vi "Initialize.vi"(8 "error in (no error)":errorcluster) -> (0 "error out":errorcluster, 3 "SGDV FPGA Target":refnum<class "SGDV FPGA Target.lvclass">)   [LabVIEW 2013, in "SGDV_Ctrl_v13_lib.lvlib" / "SGDV FPGA Target.lvclass"]
uses:
  SGDV FPGA Target.lvclass
  SGDV_Ctrl_Class/ctrl/Motor A Refnum.ctl
  SGDV FPGA Target.lvclass/SGDV FPGA Target.ctl
  SGDV_Ctrl_Class/SGDV_Ctrl_Class.lvclass
  SGDV_Ctrl_v13_lib.lvlib
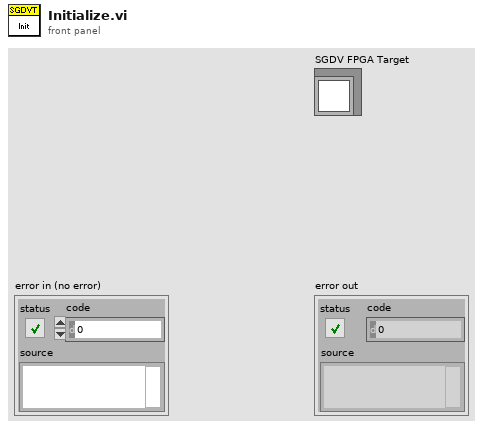
[diagram p1: front panel]
types:
  T1 = typedef "SGDV_Ctrl_v13_lib.lvlib/SGDV_Ctrl_Class.lvclass/Motor A Refnum.ctl" = cluster{"SEN":tag, "PWM":tag, "SIGN (Vel Dir)":tag, "Enc":tag, "SON":tag, "CLR":tag, "S-RDY":tag, "ALM":tag, "ALM-RST":tag, "ALO1":tag, "ALO2":tag, "ALO3":tag}
  T2 = typedef "Generic FPGA Reference.ctl" = refnum<k20>
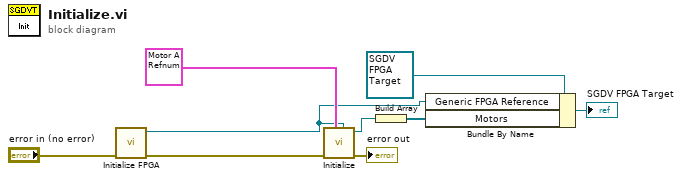
[diagram p0: block diagram]
diagram:
  n1 = call "Initialize FPGA.vi"("error in (no error)"="error in (no error)") -> ("error out"=w3:errorcluster, "Generic FPGA Reference"=w1:T2)  [unwired: 9 in]
  n2 = call "Initialize.vi"("Generic FPGA Reference"=w1, "Motor IO Refnum"=T1 {"SEN"="A/AO0", "PWM"="A/PWM0", "SIGN (Vel Dir)"="A/DIO0", "Enc"="A/ENC", "SON"="B/DIO0", "CLR"="C/DIO5", "S-RDY"="A/DIO3", "ALM"="A/DIO6", "ALM-RST"="B/DIO1", "ALO1"="B/DIO2", "ALO2"="B/DIO3", "ALO3"="B/DIO4"} ("Motor A Refnum"), "error in (no error)"=w3) -> ("error out"=→"error out":errorcluster, "SGDV_Ctrl_Class out"=w6:refnum<class "SGDV_Ctrl_Class.lvclass">)  [unwired: 7 in]
  n3 = Build Array(w6) -> (w5:refnum<class "SGDV_Ctrl_Class.lvclass">[])
  n4 = Bundle By Name(cluster=refnum<class "SGDV FPGA Target.lvclass"> refnum ("SGDV_Ctrl_v13_lib.lvlib:SGDV FPGA Target.lvclass"), "Generic FPGA Reference"=w1, "Motors"=w5) -> (→"SGDV FPGA Target":refnum<class "SGDV FPGA Target.lvclass">)
